vi "1-D Gaussian3.vi"(2 "sigma":dbl, 4 "a":dbl, 5 "x":dbl) -> (0 "y'":dbl[](array[numeric]), 1 "y":dbl)   [LabVIEW 2015]
doc: "1D Gaussian"
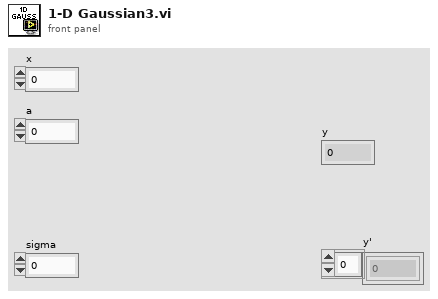
[diagram p1: front panel]
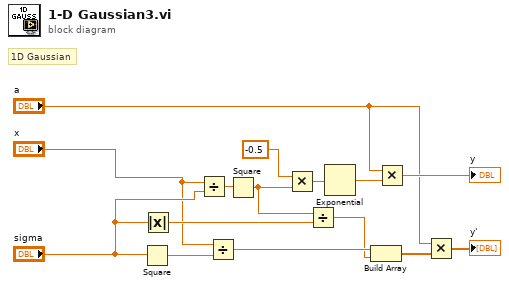
[diagram p0: block diagram]
diagram:
  # "1D Gaussian"
  n1 = Square(x="sigma") -> (x^2=w12:dbl)
  n2 = Absolute Value(x="sigma") -> (abs(x)=w7:dbl)
  n3 = Divide(x="x", y="sigma") -> (x/y=w15:dbl)
  n4 = Divide(x="x", y=w12) -> (x/y=w11:dbl)
  n5 = Square(x=w15) -> (x^2=w10:dbl)
  n6 = Multiply(x=-0.5, y=w10) -> (x*y=w13:dbl)
  n7 = Divide(x=w10, y=w7) -> (x/y=w8:dbl)
  n8 = Exponential(1:w13) -> (0:w14:dbl)
  n9 = Build Array(w11, w8) -> (w4:dbl[])
  n10 = Multiply(x="a", y=w14) -> (x*y=→"y":dbl)
  n11 = Multiply(x="a", y=w4) -> (x*y=→"y'":dbl[])
